vi "generateblock.vi"() -> (1 "wave":cdb[](array[numeric]))   [LabVIEW 2013]
uses:
  <vilib>/imath/engines/lvmath/Plug In/_Char/NIMS_CH_character datatype.ctl
  <vilib>/imath/engines/lvmath2/RunTimeEngine/ErrorHandling/NIMS_Finalize Error.vi
  <vilib>/imath/engines/lvmath2/RunTimeEngine/Managers/WorkSpace/UID Generator.vi
  <vilib>/imath/engines/lvmath/Plug In/_Char/NIMS_CH_Character RV to String.vi
  <vilib>/imath/engines/lvmath2/RunTimeEngine/Managers/SymbolTable/Clear UID.vi
  <vilib>/imath/engines/lvmath2/RunTimeEngine/NodeEndStatement/NIMS_NodeEndStatement_Output.vi
  <instcachedir>/0/NIMS_NodeEndStatement_Output_53EC0D466D134D7ABD903AC30B43404B.lvgen/NIMS_NodeEndStatement_Output_53EC0D466D134D7ABD903AC30B43404B_008.vi
  <vilib>/imath/engines/lvmath2/RunTimeEngine/BuiltInFunctions/numelements/NIMS_numelements.vi
  <instcachedir>/0/NIMS_numelements_A776DA77F73142F68C2F209B523114C5.lvgen/NIMS_numelements_A776DA77F73142F68C2F209B523114C5_001.vi
  <vilib>/imath/engines/lvmath2/RunTimeEngine/RunTimeType/NIMS_RunTimeType_From StrictType (excl LVString).vi
  <instcachedir>/0/NIMS_RunTimeType_From StrictType (excl LVString)_4DEE718D6EB74582AA20236969C084FC.lvgen/NIMS_RunTimeType_From StrictType (excl LVString)_4DEE718D6EB74582AA20236969C084FC_000.vi
  <vilib>/imath/engines/lvmath2/RunTimeEngine/LocalVariableDefStatement/MC_LocalVariableDefStatement_Display.vi
  <vilib>/imath/engines/lvmath/Plug In/_Char/NIMS_CH_String to Character Array.vi
  <vilib>/imath/engines/lvmath2/RunTimeEngine/RangeToken/NIMS_Range_R3 - Integer.vi
  <instcachedir>/0/NIMS_Range_R3 - Integer_61C6A1A9DF45400FA53C335A664ED8E6.lvgen/NIMS_Range_R3 - Integer_61C6A1A9DF45400FA53C335A664ED8E6_000.vi
  <vilib>/imath/engines/lvmath2/RunTimeEngine/NodeEndStatement/NIMS_NodeEndStatement_Get Vector.vi
  <instcachedir>/0/NIMS_NodeEndStatement_Get Vector_BE4364D373AE46158CA0B14DEB6F98C8.lvgen/NIMS_NodeEndStatement_Get Vector_BE4364D373AE46158CA0B14DEB6F98C8_003.vi
  <instcachedir>/0/NIMS_NodeEndStatement_Output_53EC0D466D134D7ABD903AC30B43404B.lvgen/NIMS_NodeEndStatement_Output_53EC0D466D134D7ABD903AC30B43404B_000.vi
  <vilib>/imath/engines/lvmath2/RunTimeEngine/CommandStatement/MC_CommandStatement_break.vi
  <vilib>/imath/engines/lvmath2/RunTimeEngine/IndexRead/NIMS V(S).vi
  <instcachedir>/0/NIMS V(S)_0488751826AF41519A22953C041130DC.lvgen/NIMS V(S)_0488751826AF41519A22953C041130DC_004.vi
  <vilib>/imathl/engines/lvmath/Functions/Error Handling/Create Error.vi
  <vilib>/imath/engines/lvmath2/RunTimeEngine/IndexReplace/NIMS M(S)=S.vi
  <instcachedir>/0/NIMS M(S)=S_4E994C4915F64874B0A495BA8935E304.lvgen/NIMS M(S)=S_4E994C4915F64874B0A495BA8935E304_001.vi
  <instcachedir>/0/NIMS_NodeEndStatement_Output_53EC0D466D134D7ABD903AC30B43404B.lvgen/NIMS_NodeEndStatement_Output_53EC0D466D134D7ABD903AC30B43404B_005.vi
  <vilib>/imath/engines/lvmath2/RunTimeEngine/RangeToken/NIMS_Range.vi
  <instcachedir>/0/NIMS_Range_7481B155BEE341ECA0F59DDB444E2C09.lvgen/NIMS_Range_7481B155BEE341ECA0F59DDB444E2C09_000.vi
  <vilib>/imath/engines/lvmath2/RunTimeEngine/IndexRead/NIMS V(R2).vi
  <instcachedir>/0/NIMS V(R2)_C76619605A0E4E9F8B2FA9389712AC47.lvgen/NIMS V(R2)_C76619605A0E4E9F8B2FA9389712AC47_000.vi
  <vilib>/imath/engines/lvmath2/RunTimeEngine/BuiltInFunctions/mirrorh/NIMS_mirrorh(GRowV).vi
  <instcachedir>/0/NIMS_mirrorh(GRowV)_B6A8CC4EAFBA4F9A82A59460D67BDFF0.lvgen/NIMS_mirrorh(GRowV)_B6A8CC4EAFBA4F9A82A59460D67BDFF0_000.vi
  <vilib>/imath/engines/lvmath2/RunTimeEngine/ErrorHandling/NIMS_Create Error From Enums.vi
  <vilib>/imath/engines/lvmath2/RunTimeEngine/ArithmeticOperatorToken/NIMS_ArithmeticOperator_times.vi
  <instcachedir>/0/NIMS_ArithmeticOperator_times_F6527734CE75451889337B8CE94765C6.lvgen/NIMS_ArithmeticOperator_times_F6527734CE75451889337B8CE94765C6_000.vi
  <vilib>/imath/engines/lvmath2/RunTimeEngine/ArithmeticOperatorToken/NIMS_ArithmeticOperator_plus.vi
  <instcachedir>/0/NIMS_ArithmeticOperator_plus_8A46DAFC24D445C9B2C97B626139369E.lvgen/NIMS_ArithmeticOperator_plus_8A46DAFC24D445C9B2C97B626139369E_004.vi
  <vilib>/imath/engines/lvmath2/RunTimeEngine/ArithmeticOperatorToken/NIMS_ArithmeticOperator_rightdiv.vi
  <instcachedir>/0/NIMS_ArithmeticOperator_rightdiv_C75411BD8BC84A93B6F1C8DA359A92EC.lvgen/NIMS_ArithmeticOperator_rightdiv_C75411BD8BC84A93B6F1C8DA359A92EC_000.vi
  <vilib>/imath/engines/lvmath2/RunTimeEngine/BuiltInFunctions/length/NIMS_length(GV).vi
  <instcachedir>/0/NIMS_length(GV)_08A3D13377FD4E4B96F5795FBF3698FA.lvgen/NIMS_length(GV)_08A3D13377FD4E4B96F5795FBF3698FA_001.vi
  <vilib>/imath/engines/lvmath2/RunTimeEngine/BuiltInFunctions/zeros/NIMS_M=zeros(I32,I32).vi
  <vilib>/imath/engines/lvmath2/RunTimeEngine/MatrixToken/NIMS_MatrixToken_RV_M.vi
  <instcachedir>/0/NIMS_MatrixToken_RV_M_82D5EDCBDBF547ADBE4B3C3DC0332972.lvgen/NIMS_MatrixToken_RV_M_82D5EDCBDBF547ADBE4B3C3DC0332972_001.vi
  <vilib>/imath/engines/lvmath2/RunTimeEngine/IndexRead/NIMS M($).vi
  <instcachedir>/0/NIMS M($)_82D1177398184AFB96A6AFB63C3C3F57.lvgen/NIMS M($)_82D1177398184AFB96A6AFB63C3C3F57_004.vi
  <vilib>/imath/engines/lvmath2/RunTimeEngine/BuiltInFunctions/conv/NIMS_conv(V,V).vi
  <instcachedir>/0/NIMS_conv(V,V)_D3E194F2B5174935BB2368CEB7AAC5A9.lvgen/NIMS_conv(V,V)_D3E194F2B5174935BB2368CEB7AAC5A9_000.vi
  <vilib>/imath/engines/lvmath2/RunTimeEngine/ErrorHandling/NIMS_Error From Error Code.vi
  <instcachedir>/0/NIMS_numelements_A776DA77F73142F68C2F209B523114C5.lvgen/NIMS_numelements_A776DA77F73142F68C2F209B523114C5_003.vi
  <vilib>/imath/engines/lvmath/Plug In/_Char/NIMS_CH_Character 1D to U8 1D.vi
  <vilib>/imath/engines/lvmath2/RunTimeEngine/BuiltInFunctions/plot/NIMS_plot(G, Arb).vi
  <instcachedir>/0/NIMS_plot(G, Arb)_C3943409FB664E118D06A85D9C4CA97C.lvgen/NIMS_plot(G, Arb)_C3943409FB664E118D06A85D9C4CA97C_000.vi
  <vilib>/imath/engines/lvmath2/RunTimeEngine/BuiltInFunctions/hold/NIMS_hold(Enums).vi
  <vilib>/imath/engines/lvmath2/RunTimeEngine/BuiltInFunctions/imag/NIMS_imag(Complex).vi
  <instcachedir>/0/NIMS_imag(Complex)_3180D40D00C843A49C2B33397F857BF3.lvgen/NIMS_imag(Complex)_3180D40D00C843A49C2B33397F857BF3_002.vi
  <vilib>/imath/engines/lvmath2/RunTimeEngine/Managers/SymbolTable/NIMS_WorkSpace.lvlib
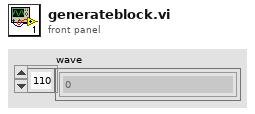
[diagram p1: front panel]
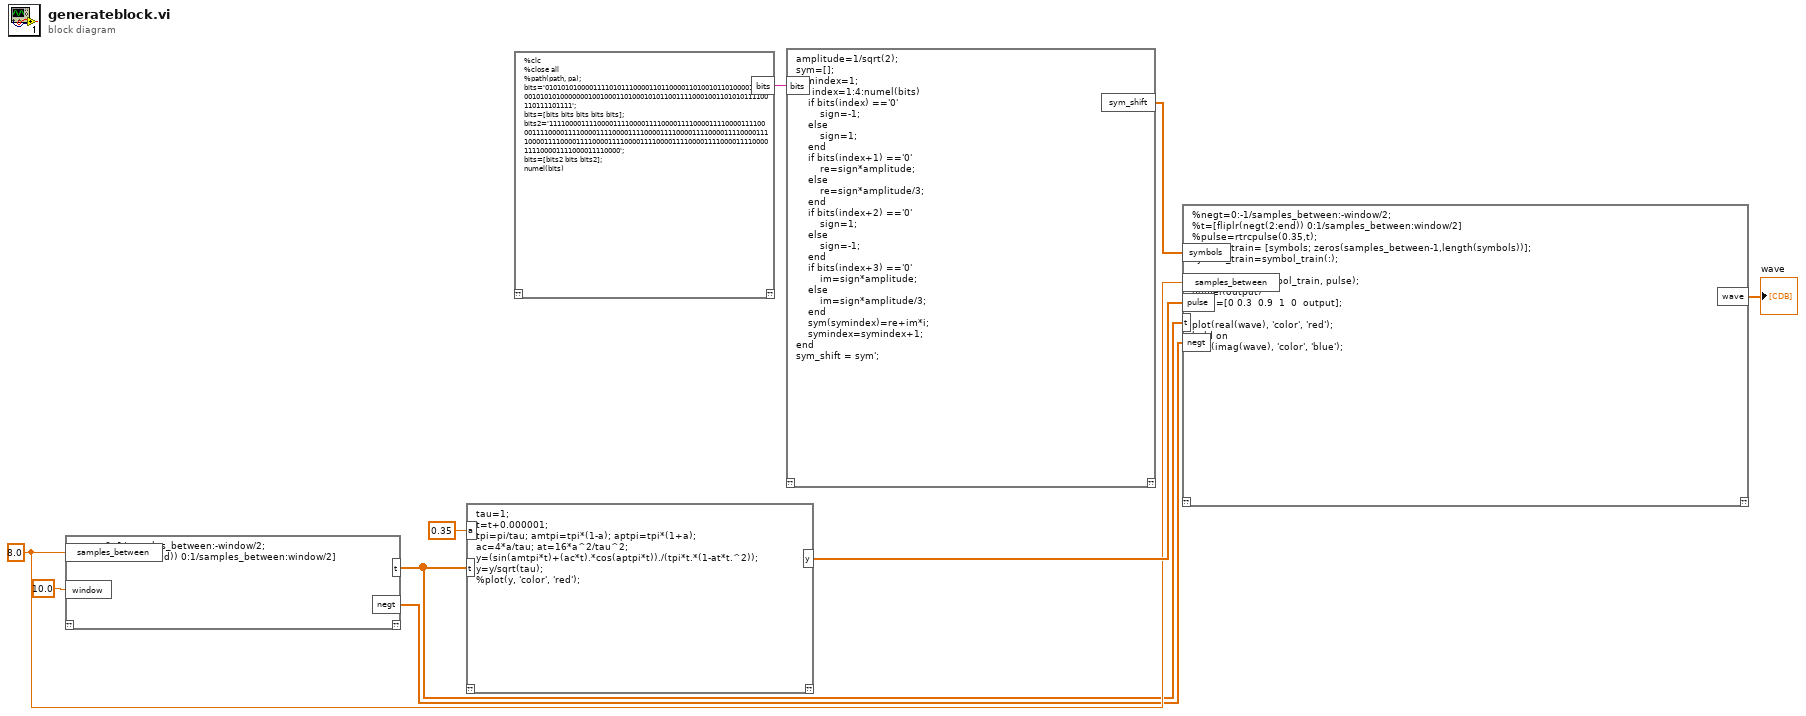
[diagram p0: block diagram]
diagram:
  w6 = 8.0 ("samples_between")
  n1 = mathscript code="negt=0:-1/samples_between:-window/2;\nt=[fliplr(negt(2:end)) 0:1/samples_between:window/2]"("samples_between"=w6, "window"=10.0) -> ("t"=w4:dbl[], "negt"=w5:dbl[])  [unwired: 1 in, 1 out]
  n2 = mathscript code="tau=1;\nt=t+0.000001;\ntpi=pi/tau; amtpi=tpi*(1-a); aptpi=tpi*(1+a);\nac=4*a/tau; at=16*a^2/tau^2;\ny=(sin(amtpi*t)+(ac*t).*cos(aptpi*t))./(tpi*t.*(1-at*t.^2));\ny=y/sqrt(tau);\n%plot(y, 'color', 'red');"("a"=0.35, "t"=w4) -> ("y"=w8:cdb[])  [unwired: 1 in, 1 out]
  n3 = mathscript code="%clc\n%close all\n%path(path, pa);\nbits='01010101000011110101110000110110000110100101101000011100010101010000000100100011010001010110011110001001101010111100110111101111';\nbits=[bits bits bits bits bits];\nbits2='11110000111100001111000011110000111100001111000011110000111100001111000011110000111100001111000011110000111100001111000011110000111100001111000011110000111100001111000011110000111100001111000011110000';\nbits=[bits2 bits bits2];\nnumel(bits)"() -> ("bits"=w1:string)  [unwired: 1 in, 1 out]
  n4 = mathscript code="amplitude=1/sqrt(2);\nsym=[];\nsymindex=1;\nfor index=1:4:numel(bits)\n    if bits(index) =='0'\n        sign=-1;\n    else\n        sign=1;\n    end\n    if bits(index+1) =='0'\n        re=sign*amplitude;\n    else\n        re=sign*amplitude/3;\n    end\n    if bits(index+2) =='0'\n        sign=1;\n    else\n        sign=-1;\n    end\n    if bits(index+3) =='0'\n        im=sign*amplitude;\n    else\n        im=sign*amplitude/3;\n    end\n    sym(symindex)=re+im*i;\n    symindex=symindex+1;\nend\nsym_shift = sym';"("bits"=w1) -> ("sym_shift"=w9:cdb[])  [unwired: 1 in, 1 out]
  n5 = mathscript code="%negt=0:-1/samples_between:-window/2;\n%t=[fliplr(negt(2:end)) 0:1/samples_between:window/2]\n%pulse=rtrcpulse(0.35,t);\nsymbol_train= [symbols; zeros(samples_between-1,length(symbols))];\nsymbol_train=symbol_train(:);\n\noutput=conv(symbol_train, pulse);\nnumel(output)\nwave=[0 0.3  0.9  1  0  output];\n\nplot(real(wave), 'color', 'red');\nhold on\nplot(imag(wave), 'color', 'blue');"("symbols"=w9, "samples_between"=w6, "pulse"=w8, "t"=w4, "negt"=w5) -> ("wave"=→"wave":cdb[])  [unwired: 1 in, 1 out]
